vi "CreateExitEvent__slk_QSM-PC (String).vi"() -> (1 "user event out":refnum<user-event>, 3 "event registration refnum out":refnum<event-registration>)   [LabVIEW 2016, in "QSM-PC (String).lvlib"]
doc: "Generates <b>Exit</b> user event for QSM-PC structure."
uses:
  Library/QSM-PC (String).lvlib
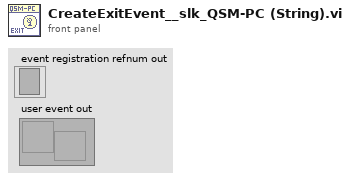
[diagram p1: front panel]
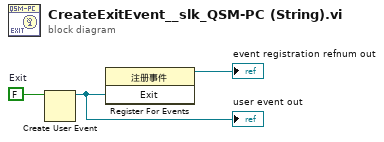
[diagram p0: block diagram]
diagram:
  w1 = FALSE  # Exit
  n1 = Create User Event(user event datatype=w1) -> (user event=w2:refnum<user-event>)  [unwired: 1 in, 1 out]
  "user event out" <- w2
  n2 = register-events(w2) -> (reference out=→"event registration refnum out":refnum<event-registration>)  [unwired: 2 in, 1 out]
